vi "close usb.vi"   [LabVIEW 2013, in "libusvlv.lvlib"]
doc: "extern \"C\" void _declspec_dll_use close_usb();"
uses:
  libusvlv.lvlib
  UsbCom.dll
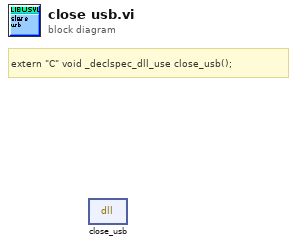
[diagram p0: block diagram]
diagram:
  # "extern \"C\" void _declspec_dll_use close_usb();"
  n1 = dll-call lib="E:/libusvlv/UsbCom.dll" fn="close_usb"() -> ()  [unwired: 3 in, 3 out]
